vi "LimitProperties.vi"(1 "State In":T1) -> (0 "State Out":T1)   [LabVIEW 2017]
uses:
  <vilib>/Platform/storage/lvStorage.llb/_stateInfoWriteProps.ctl
  <vilib>/Platform/storage/lvStorage.llb/dataStorageParams.ctl
  <vilib>/Platform/storage/lvStorage.llb/_selectedProp.ctl
  <vilib>/Platform/storage/lvStorage.llb/dataModel.ctl
  <vilib>/Platform/storage/Storage.llb/usiTypeDef.ctl
  <vilib>/Platform/storage/Storage.llb/usiPropDef.ctl
  <vilib>/express/express shared/ex_EditUserDefinedProperties/usiDataType.ctl
  <vilib>/Platform/storage/Storage.llb/specialProperties.ctl
  <vilib>/Platform/storage/Storage.llb/usiOverwriteOptions.ctl
  <vilib>/Platform/storage/lvStorage.llb/TerminalDef.ctl
  <vilib>/Platform/storage/lvStorage.llb/_TerminalStyle.ctl
  <vilib>/Utility/XNodeSupport.llb/XRect32.ctl
  <vilib>/Platform/storage/Storage.llb/usiSequenceRepresentation.ctl
  <vilib>/Platform/storage/lvStorage.llb/channelType.ctl
  <vilib>/Platform/storage/lvStorage.llb/_dataTerminals.ctl
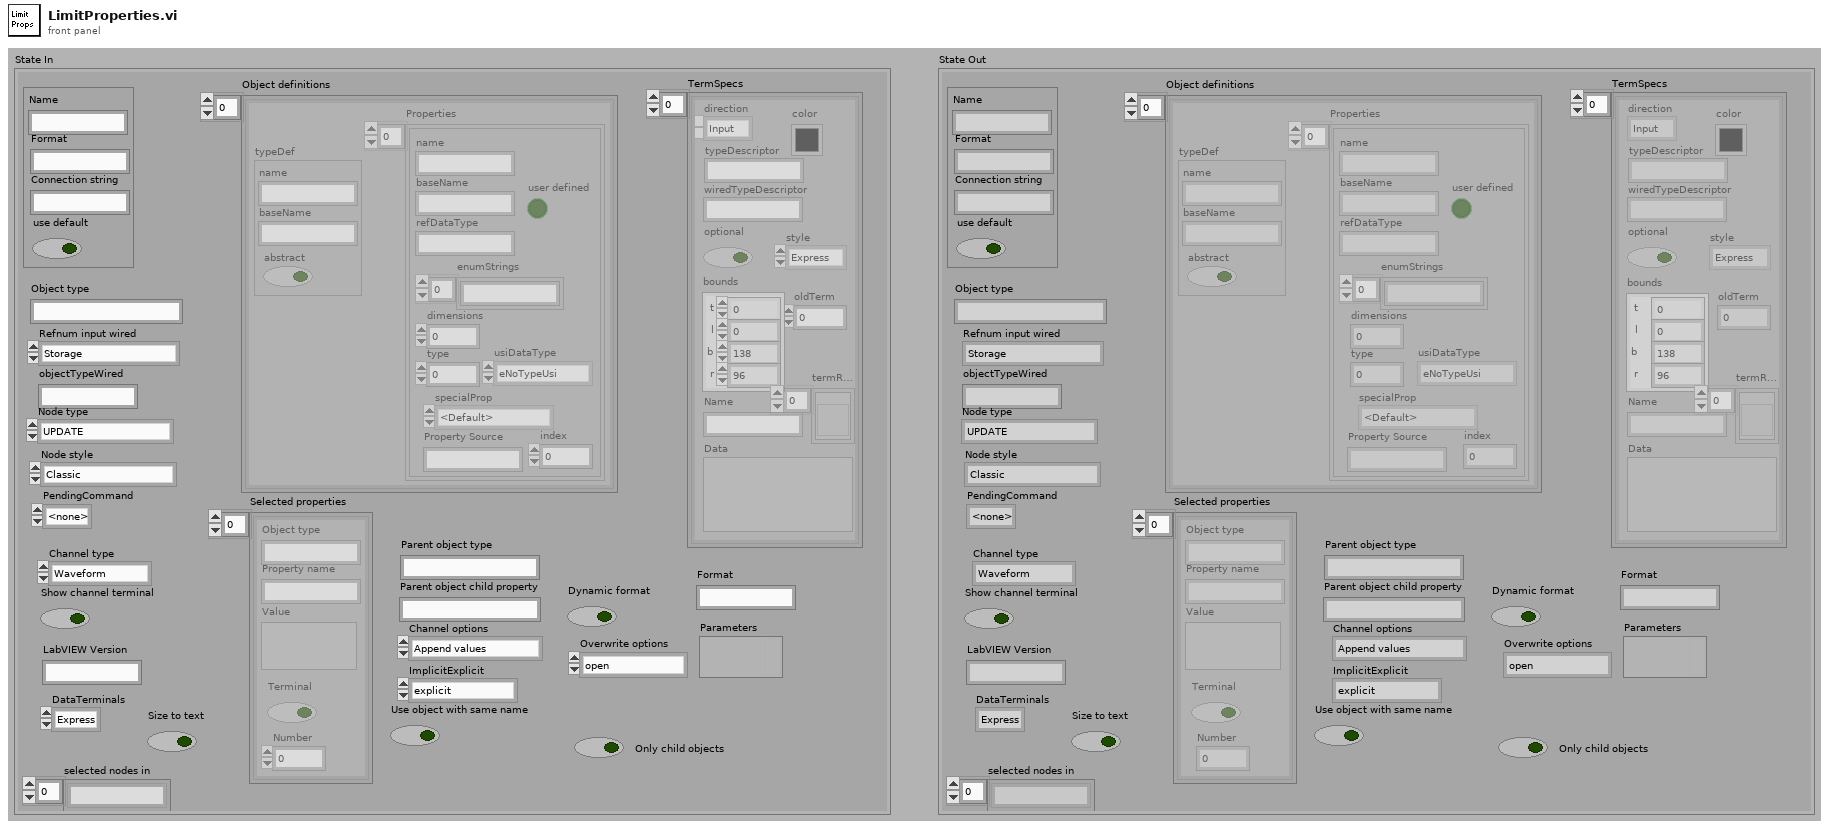
[diagram p1: front panel]
types:
  T1 = typedef "_stateInfoWriteProps.ctl" = cluster{"Data storage parameters":T2, "Object type":string, "Selected properties":T3[], "Object definitions":T4[], "Refnum input wired":enum16{"Storage", "Generic object", "Typed object", "<none>"}, "Parent object type":string, "Parent object child property":string, "Channel options":T9, "PendingCommand":enum16{"<none>", "SelPopUp", "Init"}, "Node style":enum16{"Classic", "Express"}, "Only child objects":bool, "TermSpecs":T10[], "objectTypeWired":string, "Dynamic format":bool, "Overwrite options":enum16{"open", "open or create", "create or replace", "create", "open (read only)"}, "Parameters":variant, "Format":string, "Node type":enum16{"UPDATE", "READ", "QUERY", "CREATE CHILD", "CREATE", "CONNECT", "DISCONNECT"}, "ImplicitExplicit":T13, "Channel type":T14, "Use object with same name":bool, "Show channel terminal":bool, "LabVIEW Version":string, "DataTerminals":T15, "Size to text":bool, "selected nodes in":string[]}
  T2 = typedef "dataStorageParams.ctl" = cluster{"Name":string, "Format":string, "Connection string":string, "use default":bool}
  T3 = typedef "_selectedProp.ctl" = cluster{"Object type":string, "Property name":string, "Value":variant, "Terminal":bool, "Number":i32}
  T4 = typedef "dataModel.ctl" = cluster{"typeDef":T5, "Properties":T6[]}
  T5 = typedef "usiTypeDef.ctl" = cluster{"name":string, "baseName":string, "abstract":bool}
  T6 = typedef "usiPropDef.ctl" = cluster{"name":string, "baseName":string, "refDataType":string, "dimensions":i32, "type":i32, "user defined":bool, "enumStrings":string[], "usiDataType":T7, "specialProp":T8, "Property Source":string, "index":i32}
  T7 = typedef "usiDataType.ctl" = enum16{"eNoTypeUsi", "eInt8Usi", "eInt16Usi", "eInt32Usi", "eInt64Usi", "eUInt8Usi", "eUInt16Usi", "eUInt32Usi", "eUInt64Usi", "eFloat32Usi", "eFloat64Usi", "- 0", "- 1", "- 2", "- 3", "- 4", "- 5", "- 6", "- 7", "- 8", "- 9", "eString8Usi", "eString16Usi", "eStringUsi", "eEnumUsi", "- 10", "- 11", "- 12", "- 13", "- 14", "eTimeUsi", "- 15", "- 16", "- 17", "- 18", "- 19", "- 20", "- 21", "- 22", "- 23", "eInstanceUsi", "eStoreUsi"}
  T8 = typedef "specialProperties.ctl" = enum16{"<Default>", "Channel Values", "AppendReplace", "ChannelFlags", "ValueFlags", "ImplicitExplicit", "InsertIndex", "ValuesCount", "ComparisonOperator", "Cluster", "DAQmx Channel"}
  T9 = typedef "usiOverwriteOptions.ctl" = enum16{"Append values", "Replace values at index", "Replace all values", "Append if timeline aligns"}
  T10 = typedef "TerminalDef.ctl" = cluster{"direction":enum16{"Input", "Output"}, "typeDescriptor":string, "color":u32, "oldTerm":i32, "style":T11, "optional":bool, "bounds":T12, "termRefs":refnum<vi>[], "Name":string, "Data":variant, "wiredTypeDescriptor":string}
  T11 = typedef "_TerminalStyle.ctl" = enum16{"Express", "Collapsed", "Internal"}
  T12 = typedef "XRect32.ctl" = cluster{"t":i32, "l":i32, "b":i32, "r":i32}
  T13 = typedef "usiSequenceRepresentation.ctl" = enum16{"explicit", "implicit"}
  T14 = typedef "channelType.ctl" = enum16{"Waveform", "Array of Double", "Array of String", "DDT", "Array of UInt8", "Array of Int16", "Array of Int32", "Array of Single", "Array of DateTime", "Array of Waveform", "none", "DateTime", "String", "Double", "Single", "UInt8", "Int16", "Int32"}
  T15 = typedef "_dataTerminals.ctl" = enum16{"Express", "Cluster"}
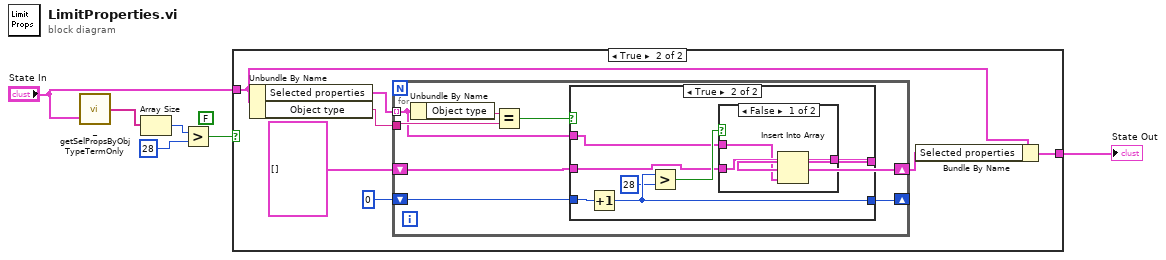
[diagram p0: block diagram]
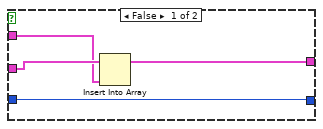
[diagram p3: hidden frame]
diagram:
  (unwired) FALSE
  n1 = call <vilib>:"_getSelPropsByObjTypeTermOnly.vi"("stateInfo"="State In") -> ("Array"=w3:string[])  [unwired: 1 in]
  n2 = Array Size(array=w3) -> (size(s)=w4:i32)
  n3 = Greater?(x=w4, y=28) -> (0:w6:bool)
  n4 = case shown="True" w6 {
    tunnel: "State In" -> [w7 w10]
    tunnel: [w7 w8] -> w2
    frame False {
    }
    frame True {
      n5 = Unbundle By Name(w10) -> ("Selected properties"=w14:T3[], "Object type"=w12:string)
      n6 = for {
        tunnel: w14 -> [w19] mode=indexing
        shift-right: [w17] -> w9
        shift-left: T3[] [] ("Selected properties") -> [w18]
        tunnel: w12 -> [w21]
        shift-right: [w15] -> _
        shift-left: 0 -> [w16]
        n7 = Unbundle By Name(w19) -> ("Object type"=w22:string)
        n8 = Equal?(x=w22, y=w21) -> (x = y?=w20:bool)
        n9 = case shown="True" w20 {
          tunnel: w19 -> [w25 w29]
          tunnel: w18 -> [w26 w28]
          tunnel: [w24 w27] -> w17
          tunnel: w16 -> [w23 w33]
          tunnel: [w23 w32] -> w15
          frame False {
            n10 = Insert Into Array(array=w26, new element=w25) -> (w24:T3[])  [unwired: 1 in]
          }
          frame True {
            n11 = Increment(x=w33) -> (x+1=w32:i32)
            n12 = Greater?(x=w32, y=28) -> (0:w30:bool)
            n13 = case shown="False" w30 {
              tunnel: w29 -> [w35 _]
              tunnel: w28 -> [w36 w37]
              tunnel: [w34 w37] -> w27
              frame False {
                n14 = Insert Into Array(array=w36, new element=w35) -> (w34:T3[])  [unwired: 1 in]
              }
              frame True {
              }
            }
          }
        }
      }
      n15 = Bundle By Name(cluster=w10, "Selected properties"=w9) -> (w8:T1)
    }
  }
  "State Out" <- w2
